vi "Sistema_3_Ejes_Cubo_CNC.vi"() -> ()   [LabVIEW 2017]
uses:
  <vilib>/Motion/Express/_s/nimc.ex.write.writeSetpoint.axis.vi
  <vilib>/Motion/Express/_s/nimc.ex.read.readExecutionData.axis.vi
  <vilib>/Motion/BlockNode/FB.NIMotion.xnode
panel:
  in  "Arreglo_Cubo 2":cluster{"X":dbl, "Y":dbl, "Z":dbl}[](array[cluster])=[{"X"=2.0, "Y"=2.0, "Z"=2.0}, {"X"=6.0, "Y"=2.0, "Z"=2.0}, {"X"=6.0, "Y"=6.0, "Z"=2.0}, {"X"=6.0, "Y"=6.0, "Z"=6.0}, {"X"=2.0, "Y"=6.0, "Z"=6.0}, {"X"=2.0, "Y"=2.0, "Z"=6.0}, {"X"=6.0, "Y"=2.0, "Z"=6.0}, {"X"=6.0, "Y"=2.0, "Z"=2.0}, {"X"=6.0, "Y"=6.0, "Z"=2.0}, {"X"=6.0, "Y"=6.0, "Z"=6.0}, {"X"=6.0, "Y"=2.0, "Z"=6.0}, {"X"=6.0, "Y"=2.0, "Z"=2.0}, {"X"=6.0, "Y"=6.0, "Z"=2.0}, {"X"=2.0, "Y"=6.0, "Z"=2.0}, {"X"=2.0, "Y"=6.0, "Z"=6.0}, {"X"=2.0, "Y"=2.0, "Z"=6.0}, {"X"=2.0, "Y"=2.0, "Z"=2.0}, {"X"=2.0, "Y"=6.0, "Z"=2.0}, {"X"=2.0, "Y"=2.0, "Z"=2.0}]
  out "3D Picture":refnum<vi>(3d-picture)
  in  "Objetos_Constantes":path=path "C:/Users/LuisFernando/Documents/UPIITA/8vo semestre/Instrumentacion Virtual Aplicada/Solidworks/Sistema_Coordenado/Archivos Blender/Archivos_constantes"
  in  "Objetos_Moviles":path=path "C:/Users/LuisFernando/Documents/UPIITA/8vo semestre/Instrumentacion Virtual Aplicada/Solidworks/Sistema_Coordenado/Archivos Blender/Archivos_moviles"
  in  "Mundo":path=path "C:/Users/LuisFernando/Documents/UPIITA/8vo semestre/Instrumentacion Virtual Aplicada/Solidworks/Sistema_Coordenado/Archivos Blender/Mundo/Mundo.wrl"
  out "EY":dbl(slide) scale=0.0..10.0
  out "EX":dbl(slide)=-0.0 scale=0.0..10.0
  out "YZ":cluster{dbl[], dbl[]}(graph)
  out "XZ":cluster{dbl[], dbl[]}(graph)
  out "Z":dbl(slide)=5.0 scale=0.0..10.0
  in  "Array 2":cluster{"X":dbl, "Y":dbl, "Z":dbl}[](array[cluster])=[{"X"=5.0, "Y"=6.5, "Z"=1.0}, {"X"=5.0, "Y"=6.5, "Z"=0.0}, {"X"=6.3225, "Y"=6.8203, "Z"=0.0}, {"X"=6.4266, "Y"=5.4635, "Z"=0.0}, {"X"=7.1399, "Y"=4.3047, "Z"=0.0}, {"X"=5.8817, "Y"=3.7865, "Z"=0.0}, {"X"=5.0, "Y"=2.75, "Z"=0.0}, {"X"=4.1183, "Y"=3.7865, "Z"=0.0}, {"X"=2.8601, "Y"=4.3047, "Z"=0.0}, {"X"=3.5734, "Y"=5.4635, "Z"=0.0}, {"X"=3.6775, "Y"=6.8203, "Z"=0.0}, {"X"=5.0, "Y"=6.5, "Z"=0.0}, {"X"=5.0, "Y"=6.5, "Z"=1.0}, {"X"=0.0, "Y"=0.0, "Z"=5.0}]
  in  "Velocidad":dbl=2.5 format="%#_13g"
  out "x > y?":bool=TRUE
  out "done":bool=TRUE
  in  "Posición Inicial":cluster{"X":dbl, "Y":dbl, "Z":dbl}={"X"=0.0, "Y"=0.0, "Z"=5.0}
  out "Paso":i32=13
  in  "Stop Button":bool
  out "EY":dbl(slide) scale=0.0..10.0
  out "EX":dbl(slide)=-0.0 scale=0.0..10.0
  out "XY":cluster{dbl[], dbl[]}(graph)
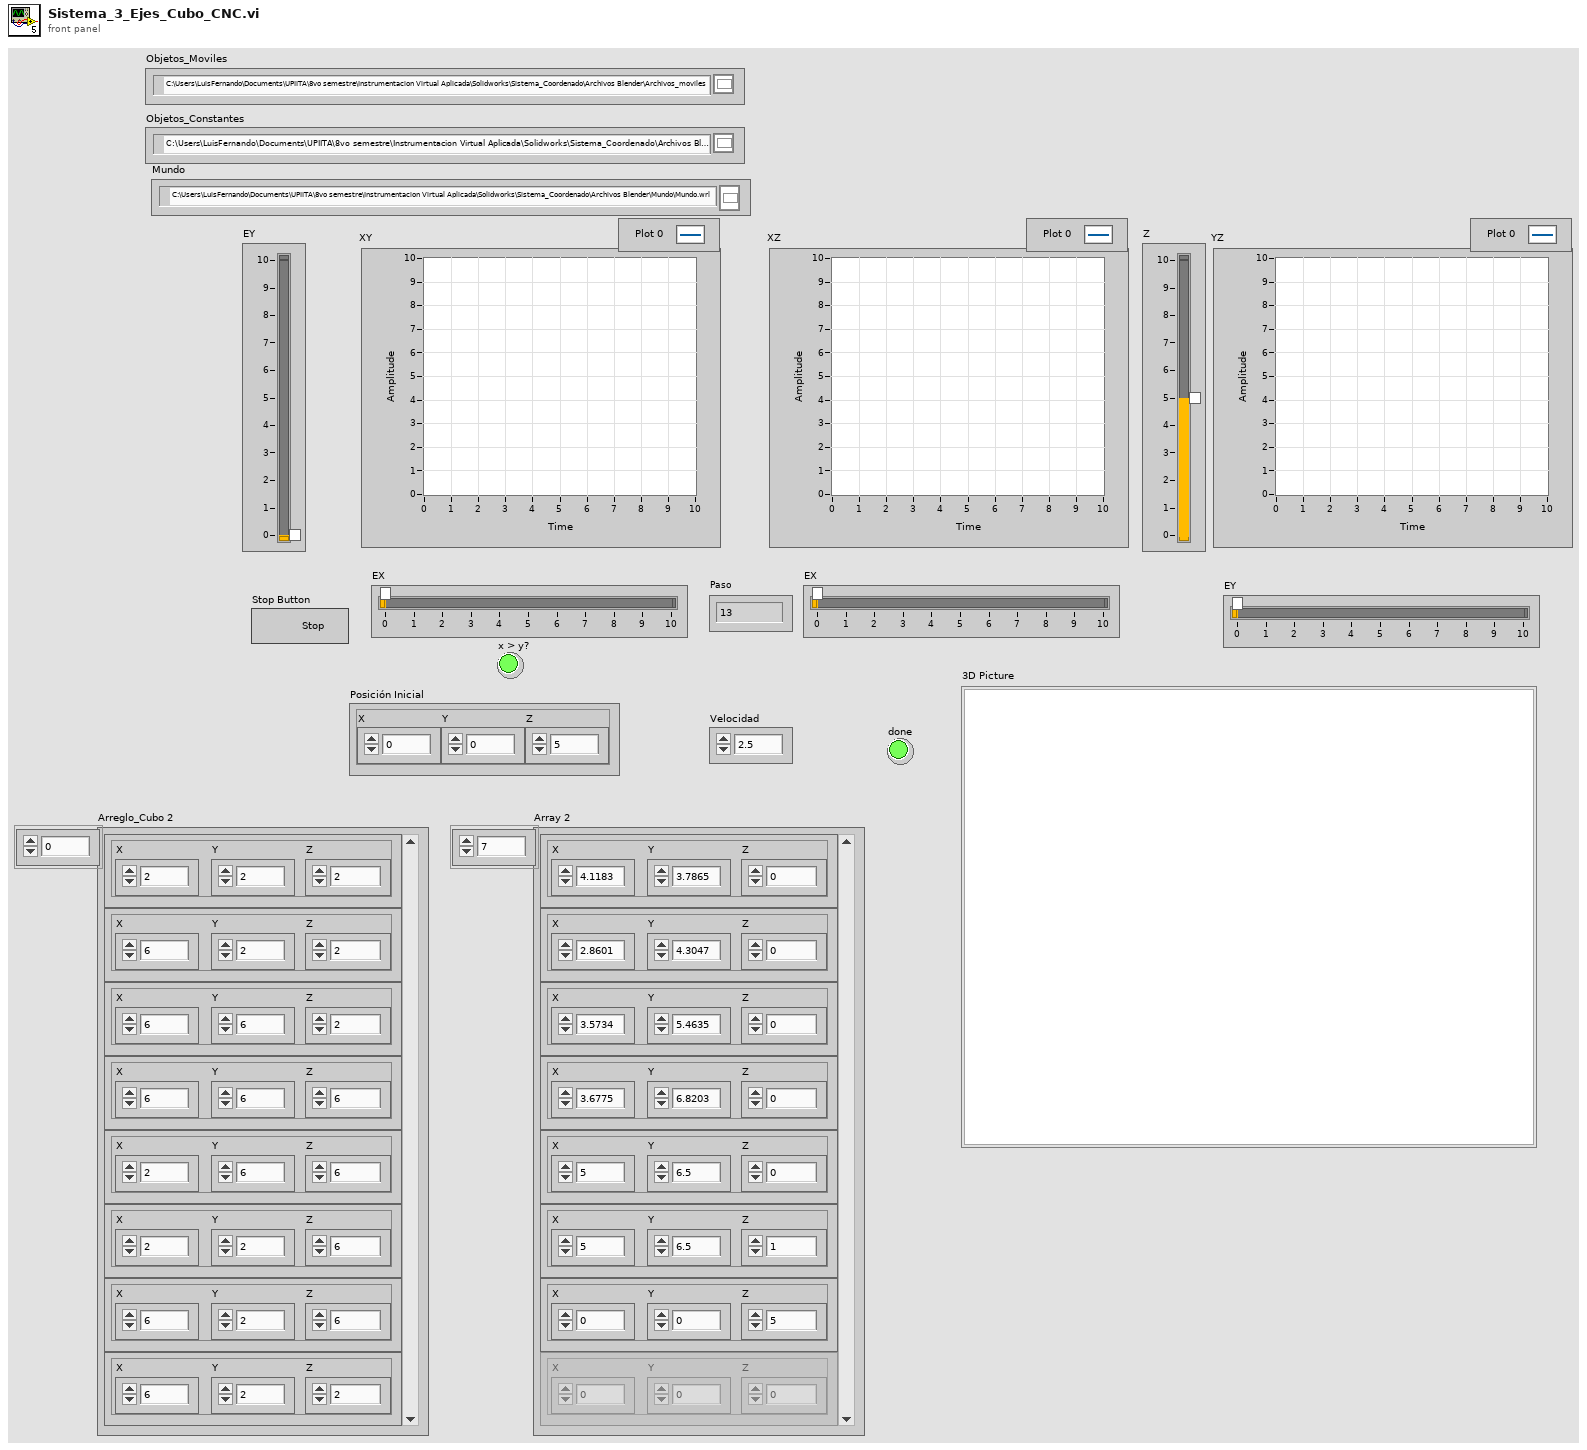
[diagram p1: front panel]
types:
  T1 = cluster{"Dif_1":dbl, "Dif_2":dbl, "Motion Resource 2":refnum<k21>, "Motion Resource 1":refnum<k21>, "Velocidad":dbl, "Posición_1":dbl, "Posición_2":dbl}
  T2 = cluster{"Motion Resource 1":refnum<k21>, "Motion Resource 2":refnum<k21>, "Motion Resource 3":refnum<k21>, "Posición_1":dbl, "Posición_2":dbl, "Posición_3":dbl, "Velocidad":dbl, "Dif_1":dbl, "Dif_2":dbl, "Dif_3":dbl}
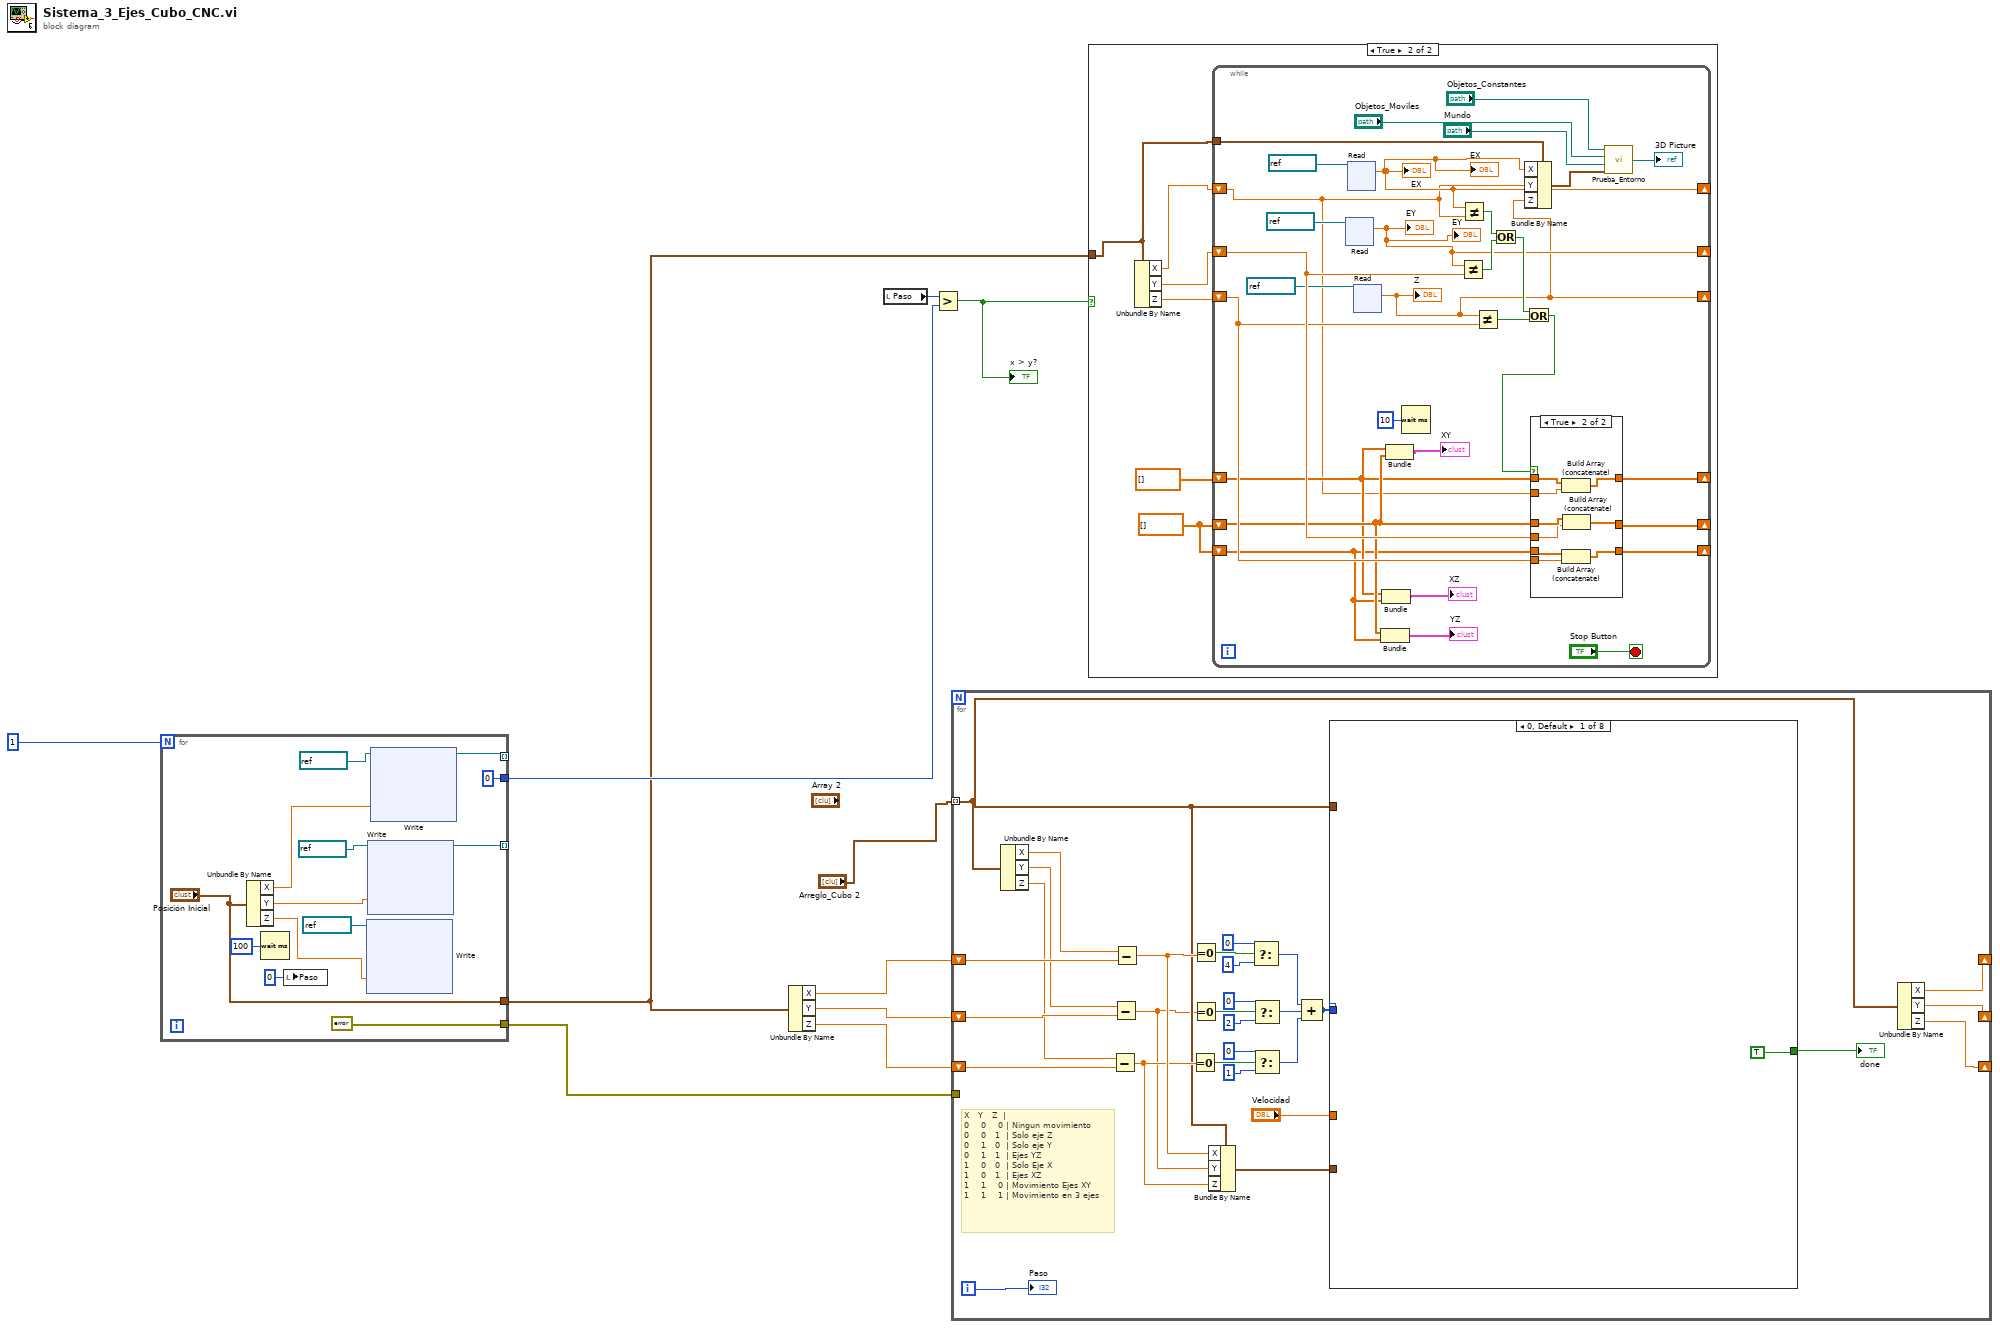
[diagram p0: block diagram]
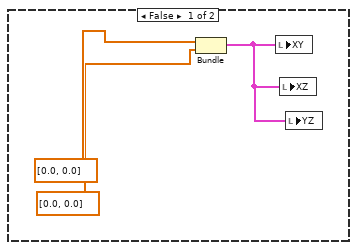
[diagram p2: hidden frame]
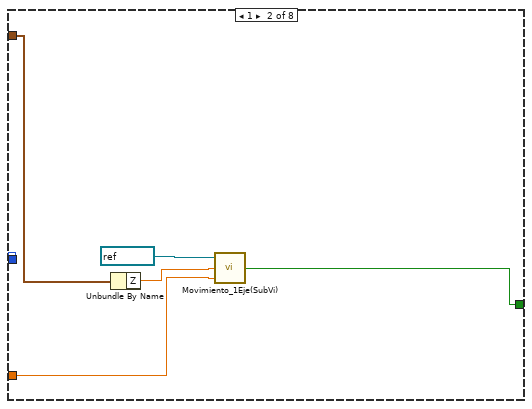
[diagram p4: hidden frame]
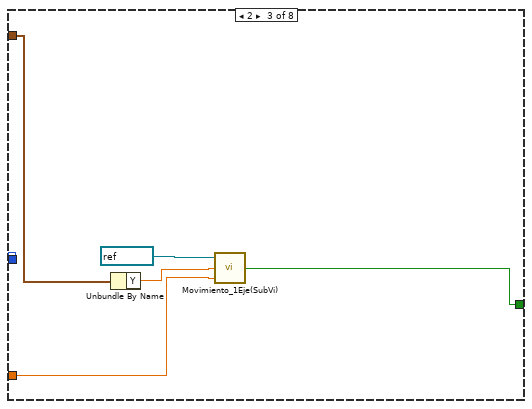
[diagram p5: hidden frame]
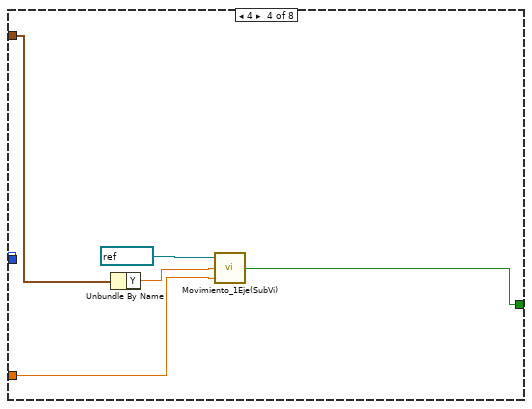
[diagram p6: hidden frame]
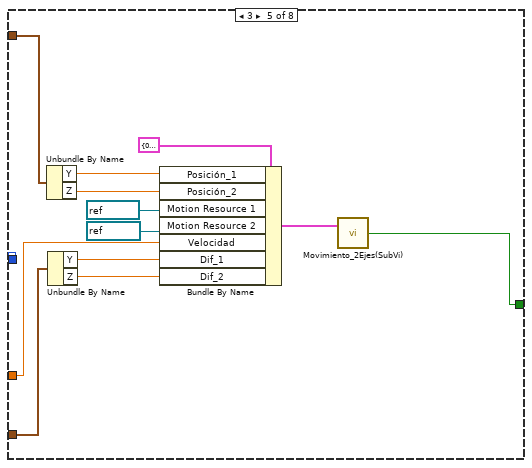
[diagram p7: hidden frame]
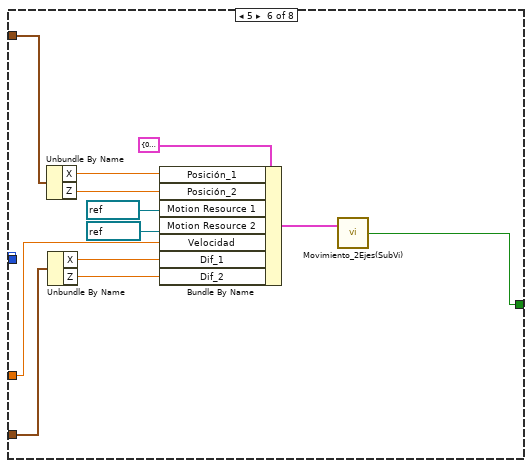
[diagram p8: hidden frame]
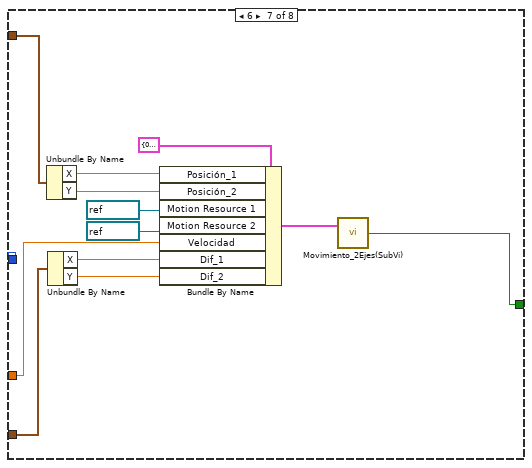
[diagram p9: hidden frame]
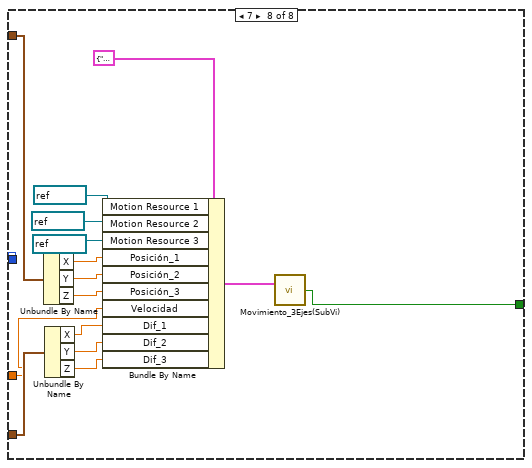
[diagram p10: hidden frame]
diagram:
  n1 = for {
    N: 1 -> [_]
    tunnel: [errorcluster {"status"=FALSE, "code"=0, "source"=""} ("error in")] -> w4
    tunnel: ["Posición Inicial"] -> w2
    tunnel: [w19] -> _ mode=indexing
    tunnel: [w18] -> _ mode=indexing
    tunnel: [0 ("y")] -> w5
    n2 = Unbundle By Name("Posición Inicial") -> ("X"=w13:dbl, "Y"=w17:dbl, "Z"=w11:dbl)
    n3 = Wait (ms)(milliseconds to wait=u32 100) -> ()  [unwired: 1 out]
    n4 = local write "Paso"(0 ("Paso")) -> ()
    n5 = xnode ("Write")("position setpoint"=w11, "resource"=refnum<k21> "EJE Z" ("Motion Resource")) -> ()  [unwired: 1 in, 2 out]
    n6 = xnode ("Write")("position setpoint"=w17, "resource"=refnum<k21> "Eje Y" ("Motion Resource")) -> ("resource out"=w19:refnum<k21>)  [unwired: 1 in, 1 out]
    n7 = xnode ("Write")("position setpoint"=w13, "resource"=refnum<k21> "Eje X" ("Motion Resource")) -> ("resource out"=w18:refnum<k21>)  [unwired: 1 in, 1 out]
  }
  n8 = Unbundle By Name(w2) -> ("X"=w9:dbl, "Y"=w8:dbl, "Z"=w3:dbl)
  n9 = local read "Paso"() -> (w7:i32)
  n10 = Greater?(x=w7, y=w5) -> (0:w6:bool)
  "x > y?" <- w6
  n11 = for {
    tunnel: "Arreglo_Cubo 2" -> [w42] mode=indexing
    tunnel: w4 -> [_]
    shift-right: [w66] -> _
    shift-left: w8 -> [w55]
    shift-right: [w67] -> _
    shift-left: w9 -> [w56]
    shift-right: [w47] -> _
    shift-left: w3 -> [w54]
    i -> [w68]
    # "X   Y   Z  |\n0    0    0 | Ningun movimiento\n0    0   1  | Solo eje Z\n0    1   0  | Solo eje Y\n0    1   1  | Ejes YZ \n1    0   0  | Solo Eje X\n1    0   1  | Ejes XZ\n1    1    0 | Movimiento Ejes XY\n1    1    1 | Movimiento en 3 ejes"
    n12 = Unbundle By Name(w42) -> ("X"=w51:dbl, "Y"=w52:dbl, "Z"=w53:dbl)
    n13 = Subtract(x=w53, y=w54) -> (x-y=w43:dbl)
    n14 = Subtract(x=w52, y=w55) -> (x-y=w41:dbl)
    n15 = Subtract(x=w51, y=w56) -> (x-y=w44:dbl)
    n16 = Equal To 0?(x=w43) -> (x = 0?=w57:bool)
    n17 = Equal To 0?(x=w44) -> (x = 0?=w65:bool)
    n18 = Equal To 0?(x=w41) -> (x = 0?=w60:bool)
    n19 = Bundle By Name(cluster=w42, "X"=w44, "Y"=w41, "Z"=w43) -> (w40:cluster{"X":dbl, "Y":dbl, "Z":dbl})
    n20 = Select(t=0, s=w65, f=4) -> (s? t:f=w49:i32)
    n21 = Select(t=0, s=w60, f=2) -> (s? t:f=w50:i32)
    n22 = Select(t=0, s=w57, f=1) -> (s? t:f=w48:i32)
    n23 = Compound Arithmetic op=ADD(w49, w50, w48) -> (w39:i32)
    n24 = case shown="0, Default" w39 {
      tunnel: [TRUE w70 w75 w80 w85 w97 w109 w133] -> w46
      tunnel: w42 -> [_ w73 w78 w83 w93 w105 w117 w129]
      tunnel: "Velocidad" -> [_ w71 w76 w81 w87 w99 w111 w121]
      tunnel: w40 -> [_ _ _ _ w90 w102 w114 w125]
      tunnel: w39 -> [_ _ _ _ _ _ _ _]
      frame 0, Default {
      }
      frame 1 {
        n25 = Unbundle By Name(w73) -> ("Z"=w72:dbl)
        n26 = call "Movimiento_1Eje(SubVi).vi"("Velocidad"=w71, "Posición"=w72, "Motion Resource 1"=refnum<k21> "EJE Z") -> ("Done"=w70:bool)
      }
      frame 2 {
        n27 = Unbundle By Name(w78) -> ("Y"=w77:dbl)
        n28 = call "Movimiento_1Eje(SubVi).vi"("Velocidad"=w76, "Posición"=w77, "Motion Resource 1"=refnum<k21> "Eje Y") -> ("Done"=w75:bool)
      }
      frame 4 {
        n29 = Unbundle By Name(w83) -> ("Y"=w82:dbl)
        n30 = call "Movimiento_1Eje(SubVi).vi"("Velocidad"=w81, "Posición"=w82, "Motion Resource 1"=refnum<k21> "Eje X") -> ("Done"=w80:bool)
      }
      frame 3 {
        n31 = Unbundle By Name(w93) -> ("Y"=w92:dbl, "Z"=w91:dbl)
        n32 = Unbundle By Name(w90) -> ("Y"=w89:dbl, "Z"=w88:dbl)
        n33 = Bundle By Name(cluster=T1 {"Dif_1"=0.0, "Dif_2"=0.0, "Motion Resource 2"="Eje Y", "Motion Resource 1"="Eje X", "Velocidad"=0.0, "Posición_1"=0.0, "Posición_2"=0.0} ("Cluster"), "Posición_1"=w92, "Posición_2"=w91, "Motion Resource 1"=refnum<k21> "Eje Y" ("Motion Resource 2"), "Motion Resource 2"=refnum<k21> "EJE Z" ("Motion Resource 1"), "Velocidad"=w87, "Dif_1"=w89, "Dif_2"=w88) -> (w86:T1)
        n34 = call "Movimiento_2Ejes(SubVi).vi"("Cluster"=w86) -> ("Done"=w85:bool)  [unwired: 1 in]
      }
      frame 5 {
        n35 = Unbundle By Name(w105) -> ("X"=w104:dbl, "Z"=w103:dbl)
        n36 = Unbundle By Name(w102) -> ("X"=w101:dbl, "Z"=w100:dbl)
        n37 = Bundle By Name(cluster=T1 {"Dif_1"=0.0, "Dif_2"=0.0, "Motion Resource 2"="Eje Y", "Motion Resource 1"="Eje X", "Velocidad"=0.0, "Posición_1"=0.0, "Posición_2"=0.0} ("Cluster"), "Posición_1"=w104, "Posición_2"=w103, "Motion Resource 1"=refnum<k21> "Eje X" ("Motion Resource 2"), "Motion Resource 2"=refnum<k21> "EJE Z" ("Motion Resource 1"), "Velocidad"=w99, "Dif_1"=w101, "Dif_2"=w100) -> (w98:T1)
        n38 = call "Movimiento_2Ejes(SubVi).vi"("Cluster"=w98) -> ("Done"=w97:bool)  [unwired: 1 in]
      }
      frame 6 {
        n39 = Unbundle By Name(w117) -> ("X"=w116:dbl, "Y"=w115:dbl)
        n40 = Unbundle By Name(w114) -> ("X"=w113:dbl, "Y"=w112:dbl)
        n41 = Bundle By Name(cluster=T1 {"Dif_1"=0.0, "Dif_2"=0.0, "Motion Resource 2"="Eje Y", "Motion Resource 1"="Eje X", "Velocidad"=0.0, "Posición_1"=0.0, "Posición_2"=0.0} ("Cluster"), "Posición_1"=w116, "Posición_2"=w115, "Motion Resource 1"=refnum<k21> "Eje X" ("Motion Resource 2"), "Motion Resource 2"=refnum<k21> "Eje Y" ("Motion Resource 1"), "Velocidad"=w111, "Dif_1"=w113, "Dif_2"=w112) -> (w110:T1)
        n42 = call "Movimiento_2Ejes(SubVi).vi"("Cluster"=w110) -> ("Done"=w109:bool)  [unwired: 1 in]
      }
      frame 7 {
        n43 = Unbundle By Name(w129) -> ("X"=w128:dbl, "Y"=w127:dbl, "Z"=w126:dbl)
        n44 = Unbundle By Name(w125) -> ("X"=w124:dbl, "Y"=w123:dbl, "Z"=w122:dbl)
        n45 = Bundle By Name(cluster=T2 {"Motion Resource 1"="Eje X", "Motion Resource 2"="Eje Y", "Motion Resource 3"="Eje Y", "Posición_1"=0.0, "Posición_2"=0.0, "Posición_3"=0.0, "Velocidad"=0.0, "Dif_1"=0.0, "Dif_2"=0.0, "Dif_3"=0.0} ("Cluster"), "Motion Resource 1"=refnum<k21> "Eje X", "Motion Resource 2"=refnum<k21> "Eje Y", "Motion Resource 3"=refnum<k21> "EJE Z", "Posición_1"=w128, "Posición_2"=w127, "Posición_3"=w126, "Velocidad"=w121, "Dif_1"=w124, "Dif_2"=w123, "Dif_3"=w122) -> (w134:T2)
        n46 = call "Movimiento_3Ejes(SubVi).vi"("Cluster"=w134) -> ("Done"=w133:bool)  [unwired: 1 in]
      }
    }
    "done" <- w46
    n47 = Unbundle By Name(w42) -> ("X"=w67:dbl, "Y"=w66:dbl, "Z"=w47:dbl)
    "Paso" <- w68
  }
  n48 = case shown="True" w6 {
    tunnel: w2 -> [_ w139]
    frame False {
      n49 = Bundle(dbl[] [0.0, 0.0], dbl[] [0.0, 0.0]) -> (w136:cluster{dbl[], dbl[]})  [unwired: 1 in]
      n50 = local write "XY"(w136) -> ()
      n51 = local write "XZ"(w136) -> ()
      n52 = local write "YZ"(w136) -> ()
    }
    frame True {
      w143 = dbl[] []
      n53 = Unbundle By Name(w139) -> ("X"=w142:dbl, "Y"=w141:dbl, "Z"=w140:dbl)
      n54 = while {
        shift-right: [w152] -> _
        shift-left: w142 -> [w151]
        shift-right: [w154] -> _
        shift-left: w141 -> [w173]
        shift-right: [w172] -> _
        shift-left: w143 -> [w157]
        shift-right: [w171] -> _
        shift-left: dbl[] [] -> [w156]
        shift-right: [w150] -> _
        shift-left: w140 -> [w160]
        shift-right: [w161] -> _
        shift-left: w143 -> [w155]
        tunnel: w139 -> [w153]
        stop <- "Stop Button" stop-if-true
        n55 = xnode "Read"("resource"=refnum<k21> "Eje Y" ("Motion Resource")) -> ("position"=w154:dbl)  [unwired: 1 in, 6 out]
        "EY" <- w154
        "EY" <- w154
        n56 = xnode "Read"("resource"=refnum<k21> "Eje X" ("Motion Resource")) -> ("position"=w152:dbl)  [unwired: 1 in, 6 out]
        "EX" <- w152
        "EX" <- w152
        n57 = xnode "Read"("resource"=refnum<k21> "EJE Z" ("Motion Resource")) -> ("position"=w150:dbl)  [unwired: 1 in, 6 out]
        "Z" <- w150
        n58 = Bundle(w157, w155) -> (→"YZ":cluster{dbl[], dbl[]})  [unwired: 1 in]
        n59 = Bundle(w156, w155) -> (→"XZ":cluster{dbl[], dbl[]})  [unwired: 1 in]
        n60 = Bundle(w156, w157) -> (→"XY":cluster{dbl[], dbl[]})  [unwired: 1 in]
        n61 = Wait (ms)(milliseconds to wait=u32 10) -> ()  [unwired: 1 out]
        n62 = Not Equal?(x=w154, y=w173) -> (x != y?=w174:bool)
        n63 = Not Equal?(x=w152, y=w151) -> (x != y?=w175:bool)
        n64 = Not Equal?(x=w150, y=w160) -> (x != y?=w164:bool)
        n65 = Or(x=w175, y=w174) -> (x .or. y?=w163:bool)
        n66 = Bundle By Name(cluster=w153, "X"=w152, "Y"=w151, "Z"=w150) -> (w149:cluster{"X":dbl, "Y":dbl, "Z":dbl})
        n67 = Or(x=w163, y=w164) -> (x .or. y?=w162:bool)
        n68 = case shown="True" w162 {
          tunnel: w156 -> [w187 w196]
          tunnel: w157 -> [w186 w193]
          tunnel: w151 -> [_ w195]
          tunnel: w173 -> [_ w192]
          tunnel: [w186 w191] -> w172
          tunnel: [w187 w194] -> w171
          tunnel: w155 -> [w185 w190]
          tunnel: [w185 w188] -> w161
          tunnel: w160 -> [_ w189]
          frame False {
          }
          frame True {
            n69 = Build Array (concatenate)(w196, w195) -> (w194:dbl[])
            n70 = Build Array (concatenate)(w190, w189) -> (w188:dbl[])
            n71 = Build Array (concatenate)(w193, w192) -> (w191:dbl[])
          }
        }
        n72 = call "Prueba_Entorno.vi"("Posición"=w149, "Mundo"="Mundo", "Objetos_Moviles"="Objetos_Moviles", "Objetos_Constantes"="Objetos_Constantes") -> ("3D Picture"=→"3D Picture":refnum<vi>)
      }
    }
  }
